vi "ABAPI Dist Cmp Two Paths.vi"(4 "path2":path, 5 "path1":path) -> (0 "different types?":bool, 1 "relative path from 1 to 2":path, 2 "common path":path)   [LabVIEW 2020]
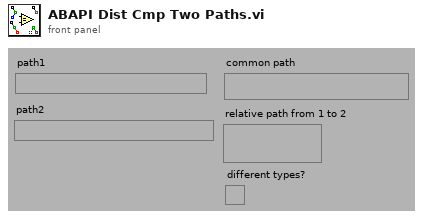
[diagram p1: front panel]
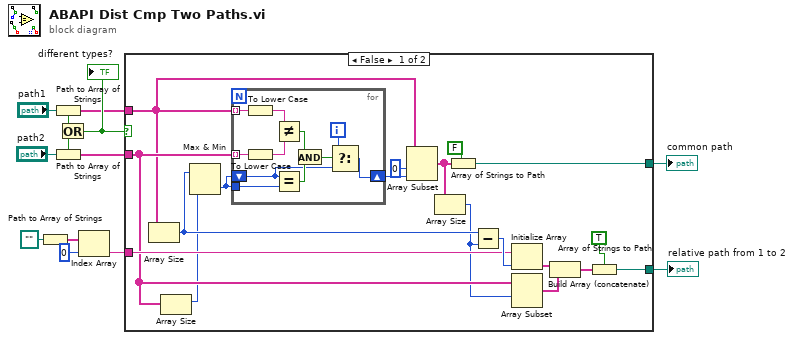
[diagram p0: block diagram]
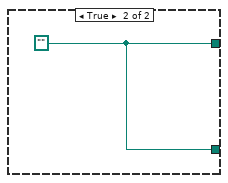
[diagram p2: hidden frame]
diagram:
  n1 = Path to Array of Strings(0:path "..") -> (2:w2:string[])  [unwired: 1 out]
  n2 = Path to Array of Strings(0:"path1") -> (1:w11:bool, 2:w8:string[])
  n3 = Path to Array of Strings(0:"path2") -> (1:w10:bool, 2:w7:string[])
  n4 = Or(x=w11, y=w10) -> (x .or. y?=w9:bool)
  "different types?" <- w9
  n5 = Index Array(array=w2, index=0) -> (element=w1:string)
  n6 = case shown="False" w9 {
    tunnel: w8 -> [w18 _]
    tunnel: w7 -> [w23 _]
    tunnel: [w28 w43] -> w6
    tunnel: [w19 w43] -> w5
    tunnel: w1 -> [w25 _]
    frame False {
      n7 = Array Size(array=w18) -> (size(s)=w17:i32)
      n8 = Array Size(array=w23) -> (size(s)=w16:i32)
      n9 = Max & Min(x=w17, y=w16) -> (min(x,y)=w15:i32)  [unwired: 1 out]
      n10 = for {
        tunnel: w18 -> [w42] mode=indexing
        tunnel: w23 -> [w41] mode=indexing
        shift-right: [w34] -> w31
        shift-left: w15 -> [w35]
        tunnel: w15 -> [w40]
        i -> [w36]
        n11 = To Lower Case(string=w42) -> (all lower case string=w33:string)
        n12 = To Lower Case(string=w41) -> (all lower case string=w32:string)
        n13 = Not Equal?(x=w33, y=w32) -> (x != y?=w38:bool)
        n14 = Equal?(x=w35, y=w40) -> (x = y?=w39:bool)
        n15 = And(x=w38, y=w39) -> (x .and. y?=w37:bool)
        n16 = Select(t=w36, s=w37, f=w35) -> (s? t:f=w34:i32)
      }
      n17 = Array Subset(array=w18, index=0, length=w31) -> (w27:string[])
      n18 = Array Size(array=w27) -> (size(s)=w14:i32)
      n19 = Array of Strings to Path(0:w27, 1:FALSE ("relative")) -> (2:w28:path)
      n20 = Subtract(x=w17, y=w14) -> (x-y=w26:i32)
      n21 = Initialize Array(w25, w26) -> (w24:string[])
      n22 = Array Subset(array=w23, index=w14) -> (w22:string[])  [unwired: 1 in]
      n23 = Build Array (concatenate)(w24, w22) -> (w21:string[])
      n24 = Array of Strings to Path(0:w21, 1:TRUE ("relative")) -> (2:w19:path)
    }
    frame True {
      w43 = path "" ("path")
    }
  }
  "relative path from 1 to 2" <- w5
  "common path" <- w6
